vi "Kernel - System Manager.vi"(7 "Data in - System Manager":T1 {"Type of Acquisition" items=["Power Analysis", "Harmonics Analysis", "Symmetrical Components Analysis"]}, 8 "error in":errorcluster, 10 "State":string, 11 "message queue":refnum<queue>) -> (0 "error out":errorcluster, 3 "message queue (out)":refnum<queue>, 4 "Stop?":bool, 5 "Data out - System Manager":T1 {"Type of Acquisition" items=["Power Analysis", "Harmonics Analysis", "Symmetrical Components Analysis"]})   [LabVIEW 2021]
uses:
  Typedefs/Data - System Manager.ctl
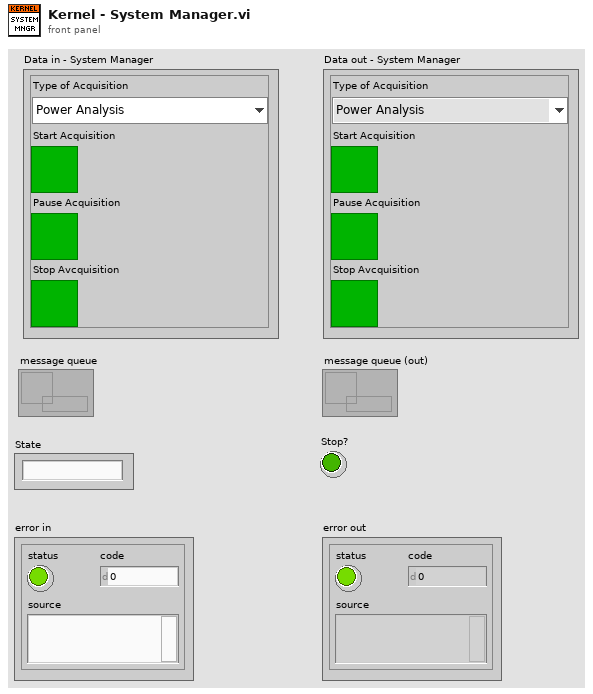
[diagram p1: front panel]
types:
  T1 = typedef "Data - System Manager.ctl" = cluster{"Stop Avcquisition":bool, "Pause Acquisition":bool, "Start Acquisition":bool, "Type of Acquisition":u16}
  T2 = cluster{"Stop Avcquisition":bool, "Pause Acquisition":bool, "Start Acquisition":bool, "Type of Acquisition":u16}
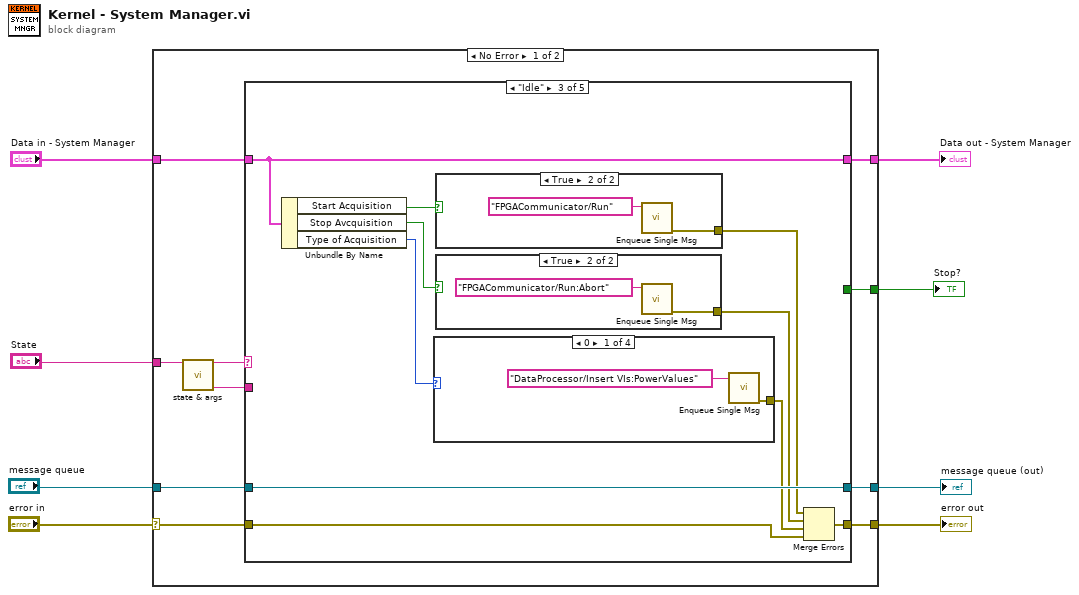
[diagram p0: block diagram]
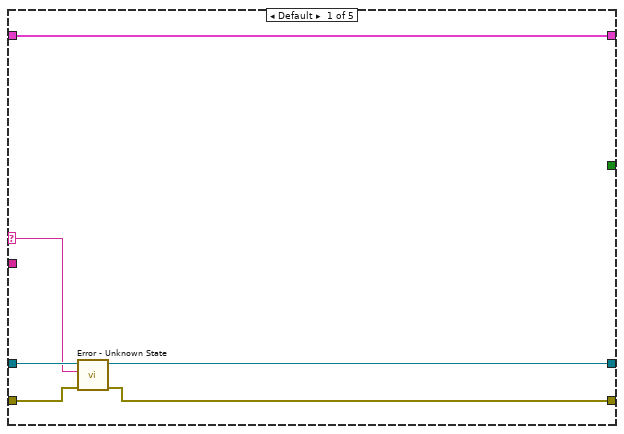
[diagram p2: hidden frame]
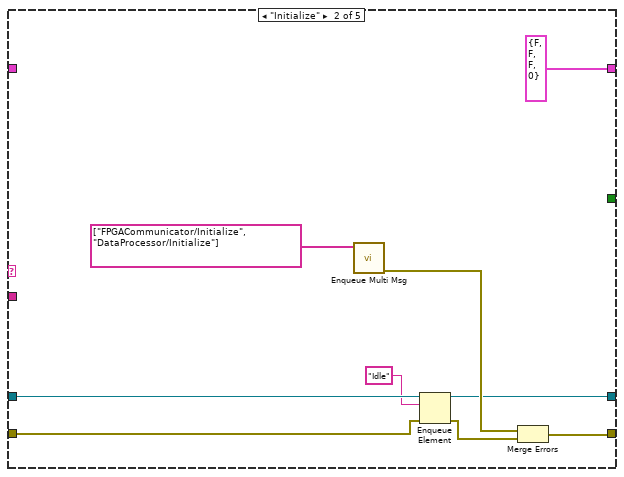
[diagram p3: hidden frame]
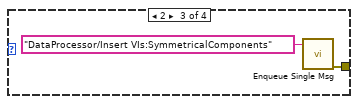
[diagram p5: hidden frame]
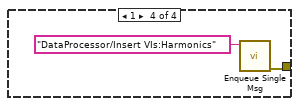
[diagram p6: hidden frame]
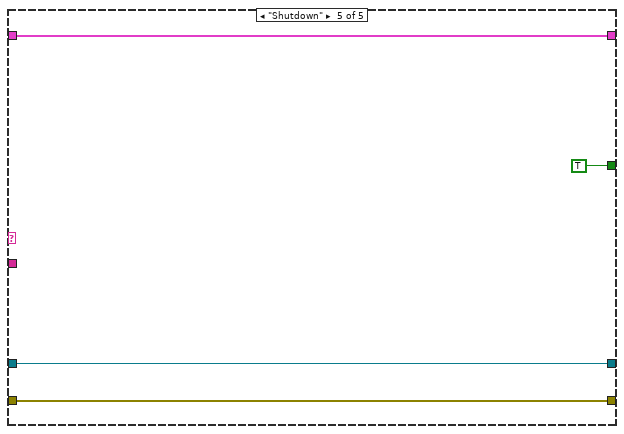
[diagram p10: hidden frame]
diagram:
  n1 = case shown="No Error" "error in" {
    selector: "error in" -> [w14 w62]
    tunnel: "State" -> [w18 _]
    tunnel: "message queue" -> [w15 w63]
    tunnel: [w13 w63] -> w5
    tunnel: [w12 w62] -> w6
    tunnel: [w11 _] -> w3
    tunnel: [w10 w61] -> w1
    tunnel: "Data in - System Manager" -> [w9 w61]
    frame No Error {
      n2 = call "state & args.vi"("state:args"=w18) -> ("args"=w16:string, "state"=w17:string)  [unwired: 9 in]
      n3 = case shown="\"Idle\"" w17 {
        selector: w17 -> [w22 _ _ _ _]
        tunnel: w16 -> [_ _ _ _ _]
        tunnel: w15 -> [w24 w28 w43 w55 w59]
        tunnel: w14 -> [w23 w29 w37 w54 w58]
        tunnel: [w21 w27 w43 w55 w59] -> w13
        tunnel: [w20 w31 w38 w54 w58] -> w12
        tunnel: [_ _ _ _ TRUE] -> w11
        tunnel: [w19 T2 {"Stop Avcquisition"=FALSE, "Pause Acquisition"=FALSE, "Start Acquisition"=FALSE, "Type of Acquisition"=0} ("Cluster") w42 w56 w57] -> w10
        tunnel: w9 -> [w19 _ w42 w56 w57]
        frame Default {
          n4 = call "Error - Unknown State.vi"("error in"=w23, "state"=w22, "queue"=w24) -> ("error out"=w20:errorcluster, "queue out"=w21:refnum<queue>)  [unwired: 7 in]
        }
        frame "Initialize" {
          n5 = call "Enqueue Multi Msg.vi"("queue/message"=string[] ["FPGACommunicator/Initialize", "DataProcessor/Initialize"]) -> ("error out"=w30:errorcluster)  [unwired: 10 in]
          n6 = Enqueue Element(queue=w28, element="Idle", error in (no error)=w29) -> (queue out=w27:refnum<queue>, error out=w26:errorcluster)  [unwired: 1 in, 1 out]
          n7 = Merge Errors(w30, w26) -> (w31:errorcluster)
        }
        frame "Idle" {
          n8 = Unbundle By Name(w42) -> ("Start Acquisition"=w41:bool, "Stop Avcquisition"=w40:bool, "Type of Acquisition"=w39:u16)
          n9 = case shown="0" w39 {
            tunnel: [w45 _ w47 w48] -> w36
            frame 0 {
              n10 = call "Enqueue Single Msg.vi"("queue/message"="DataProcessor/Insert VIs:PowerValues") -> ("error out"=w45:errorcluster)  [unwired: 10 in]
            }
            frame Default {
            }
            frame 2 {
              n11 = call "Enqueue Single Msg.vi"("queue/message"="DataProcessor/Insert VIs:SymmetricalComponents") -> ("error out"=w47:errorcluster)  [unwired: 10 in]
            }
            frame 1 {
              n12 = call "Enqueue Single Msg.vi"("queue/message"="DataProcessor/Insert VIs:Harmonics") -> ("error out"=w48:errorcluster)  [unwired: 10 in]
            }
          }
          n13 = case shown="True" w41 {
            tunnel: [_ w52] -> w34
            frame False {
            }
            frame True {
              n14 = call "Enqueue Single Msg.vi"("queue/message"="FPGACommunicator/Run") -> ("error out"=w52:errorcluster)  [unwired: 10 in]
            }
          }
          n15 = case shown="True" w40 {
            tunnel: [_ w50] -> w35
            frame False {
            }
            frame True {
              n16 = call "Enqueue Single Msg.vi"("queue/message"="FPGACommunicator/Run:Abort") -> ("error out"=w50:errorcluster)  [unwired: 10 in]
            }
          }
          n17 = Merge Errors(w34, w35, w36, w37) -> (w38:errorcluster)
        }
        frame "Error" {
        }
        frame "Shutdown" {
        }
      }
    }
    frame Error {
    }
  }
  "error out" <- w6
  "Stop?" <- w3
  "message queue (out)" <- w5
  "Data out - System Manager" <- w1
